vi "score sorter.vi"(0 "Score":i32[](array[numeric])) -> (1 "sorted ID":i32[](array[numeric]), 2 "sorted score":dbl[](array[numeric]), 3 "Students":cluster{cluster{"Score":i32[], "ID":i32[]}}[](array[cluster]))   [LabVIEW 2014]
panel:
  out "ID":i32[](array[numeric])
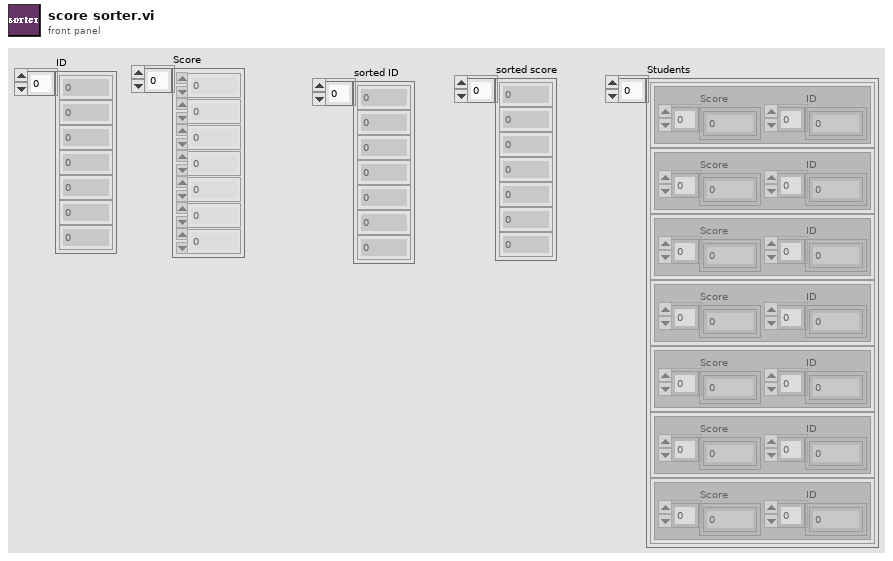
[diagram p1: front panel]
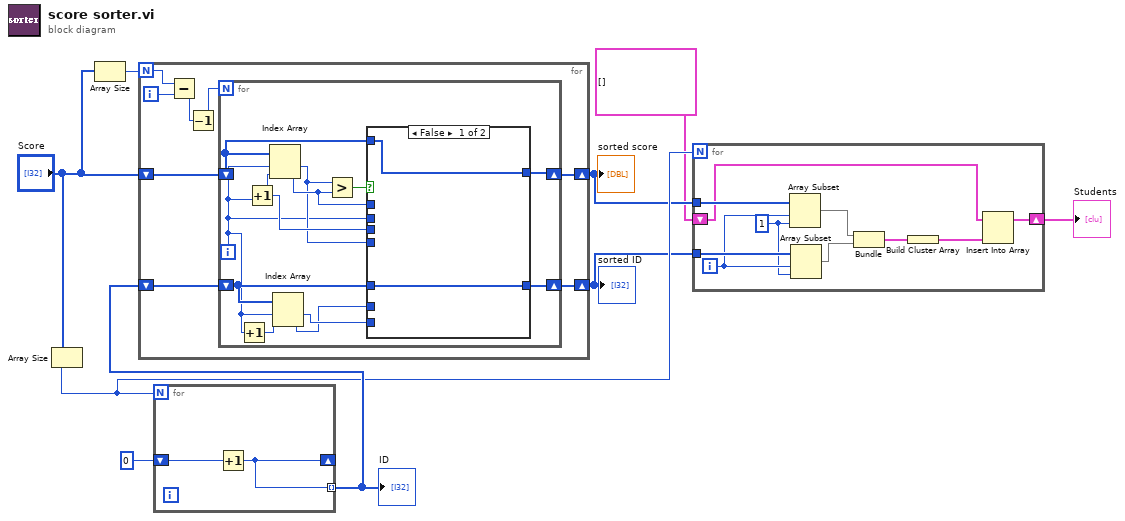
[diagram p0: block diagram]
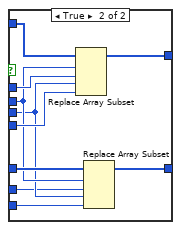
[diagram p2: hidden frame]
diagram:
  n1 = Array Size(array="Score") -> (size(s)=w5:i32)
  n2 = Array Size(array="Score") -> (size(s)=w9:i32)
  n3 = for {
    N: w5 -> [_]
    shift-right: [w10] -> _
    shift-left: 0 -> [w11]
    tunnel: [w10] -> w6 mode=indexing
    n4 = Increment(x=w11) -> (x+1=w10:i32)
  }
  "ID" <- w6
  n5 = for {
    N: w9 -> [w17]
    shift-right: [w18] -> w4
    shift-left: "Score" -> [w19]
    shift-right: [w12] -> w3
    shift-left: w6 -> [w13]
    i -> [w16]
    n6 = Subtract(x=w17, y=w16) -> (x-y=w15:i32)
    n7 = Decrement(x=w15) -> (x-1=w14:i32)
    n8 = for {
      N: w14 -> [_]
      shift-right: [w26] -> w18
      shift-left: w19 -> [w30]
      shift-right: [w25] -> w12
      shift-left: w13 -> [w24]
      i -> [w23]
      n9 = Increment(x=w23) -> (x+1=w22:i32)
      n10 = Increment(x=w23) -> (x+1=w29:i32)
      n11 = Index Array(array=w30, index #1=w23, index #2=w29) -> (element #1=w27:i32, element #2=w28:i32)
      n12 = Index Array(array=w24, index #1=w23, index #2=w22) -> (element #1=w21:i32, element #2=w20:i32)
      n13 = Greater?(x=w27, y=w28) -> (0:w31:bool)
      n14 = case shown="False" w31 {
        tunnel: w30 -> [w33 w40]
        tunnel: w23 -> [_ w37]
        tunnel: w28 -> [_ w43]
        tunnel: w29 -> [_ w36]
        tunnel: w27 -> [_ w42]
        tunnel: [w33 w41] -> w26
        tunnel: [w32 w39] -> w25
        tunnel: w24 -> [w32 w38]
        tunnel: w21 -> [_ w35]
        tunnel: w20 -> [_ w34]
        frame False {
        }
        frame True {
          n15 = Replace Array Subset(array=w40, new element #1=w43, index #1=w37, new element #2=w42, index #2=w36) -> (w41:i32[])
          n16 = Replace Array Subset(array=w38, new element #1=w34, index #1=w37, new element #2=w35, index #2=w36) -> (w39:i32[])
        }
      }
    }
  }
  "sorted score" <- w4
  "sorted ID" <- w3
  n17 = for {
    N: w5 -> [_]
    tunnel: w4 -> [w53]
    tunnel: w3 -> [w52]
    shift-right: [w45] -> w2
    shift-left: cluster{cluster{i32[], i32[]}}[] [] -> [w44]
    i -> [w51]
    w50 = 1 ("length")
    n18 = Array Subset(array=w53, index=w51, length=w50) -> (w48:i32[])
    n19 = Array Subset(array=w52, index=w51, length=w50) -> (w47:i32[])
    n20 = Bundle(w48, w47) -> (w49:cluster{i32[], i32[]})  [unwired: 1 in]
    n21 = Build Cluster Array(w49) -> (w46:cluster{cluster{i32[], i32[]}}[])
    n22 = Insert Into Array(array=w44, new element=w46) -> (w45:cluster{cluster{i32[], i32[]}}[])  [unwired: 1 in]
  }
  "Students" <- w2
